vi "Async-TCP-Serv.vi"() -> ()   [LabVIEW 2017]
panel:
  in  "Port":u16=5005
  in  "Stop Button":bool
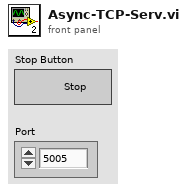
[diagram p1: front panel]
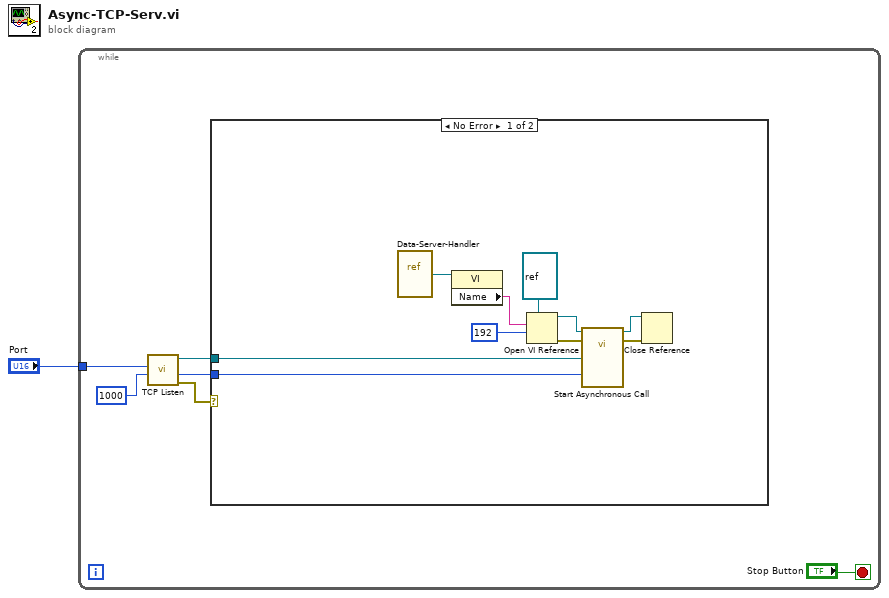
[diagram p0: block diagram]
diagram:
  n1 = while {
    tunnel: "Port" -> [w3]
    stop <- "Stop Button" stop-if-true
    n2 = call <vilib>:"TCP Listen.vi"("timeout ms (wait forever: -1)"=1000, "port"=w3) -> ("error out"=w5:errorcluster, "remote port"=w2:u16, "connection ID"=w4:refnum<k5>)  [unwired: 5 in, 2 out]
    n3 = case shown="No Error" w5 {
      tunnel: w4 -> [w9 _]
      tunnel: w2 -> [w8 _]
      frame No Error {
        n4 = vi-ref "Data-Server-Handler.vi"() -> (w15:refnum<vi>)
        n5 = property class="VI"(reference=w15) -> ("Name"=w14:string)  [unwired: 1 in, 2 out]
        n6 = Open VI Reference(type specifier VI Refnum (for type only)=refnum<vi> refnum, vi path=w14, options=192) -> (vi reference=w11:refnum<vi>, error out=w10:errorcluster)  [unwired: 3 in]
        n7 = call-by-ref "Start Asynchronous Call"(reference=w11, error in=w10, "Remote Port"=w8, "connection ID"=w9) -> (reference out=w16:refnum<vi>, error out=w17:errorcluster)  [unwired: 1 in]
        n8 = Close Reference(reference=w16, error in (no error)=w17) -> ()  [unwired: 1 out]
      }
      frame Error {
      }
    }
  }
